vi "Read Output Till Keyword.vi"(7 "timeout [ms]":u32, 8 "error in":errorcluster, 10 "keywords":string[](array[string])=["error", "USERkeyword"], 11 "GOLPI ref. in":T1={"pipe handle"={"lv_proc.dll file path"=path "", "process instance handle"=[]}, "fast read timeout [ms]"=500, "fast read settle time [ms]"=10, "fast read to multiple [ms]"=1, "max elements per input line"=100, "slow read timeout [ms]"=500}) -> (0 "error out":errorcluster, 2 "read buffer":string, 3 "GOLPI ref. out":T1={"pipe handle"={"lv_proc.dll file path"=path "", "process instance handle"=[]}, "fast read timeout [ms]"=500, "fast read settle time [ms]"=10, "fast read to multiple [ms]"=1, "max elements per input line"=100, "slow read timeout [ms]"=500}, 5 "bytes remaining":i32)   [LabVIEW 2013, in "GOLPI library.lvlib"]
doc: "Continually reads output of GNU Octave. If one of strings specified in keywords terminal is found in output, reading stops.\nIf timeout is exceeded, returns only part of buffer and returns number of bytes remaining in the stdout (if any).\nOne of keywords should be 'error' in the case error occurs, otherwise the vi will wait till timeout."
uses:
  GOLPI library.lvlib
  Private/Type Definitions/GOLPI reference Type Def.ctl
  LV Process.lvlibp/Pipe Handle.ctl
  Private/Type Definitions/Custom Error Codes Enum Type Def.vi
  LV Process.lvlibp
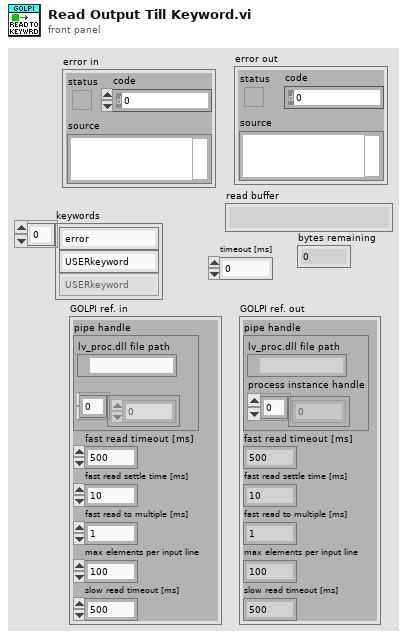
[diagram p1: front panel]
types:
  T1 = typedef "GOLPI library.lvlib/GOLPI reference Type Def.ctl" = cluster{"pipe handle":T2, "fast read timeout [ms]":u32, "fast read settle time [ms]":u32, "fast read to multiple [ms]":u32, "max elements per input line":u32, "slow read timeout [ms]":u32}
  T2 = typedef "LV Process.lvlibp/Pipe Handle.ctl" = cluster{"lv_proc.dll file path":path, "process instance handle":u32[]}
  T3 = typedef "GOLPI library.lvlib/Custom Error Codes Enum Type Def.vi" = enum16{"no error", "00 working directory PAR1 missing", "01 octave binary PAR1 missing", "02 octave report error PAR1", "03 empty output last cmd PAR1", "04 missing temporary file PAR1", "05 pwd PAR 1 not exist", "10 var PAR1 not string", "11 var PAR1 not num, scal, ~compl", "12 var PAR1 not num, scal, compl", "13 var PAR1 not num, vect, ~compl", "14 var PAR1 not num, vect, compl", "15 var PAR1 not num, mat, ~compl", "16 var PAR1 not num, mat, ~compl", "30 WARNING read timeout", "99 not finished"}
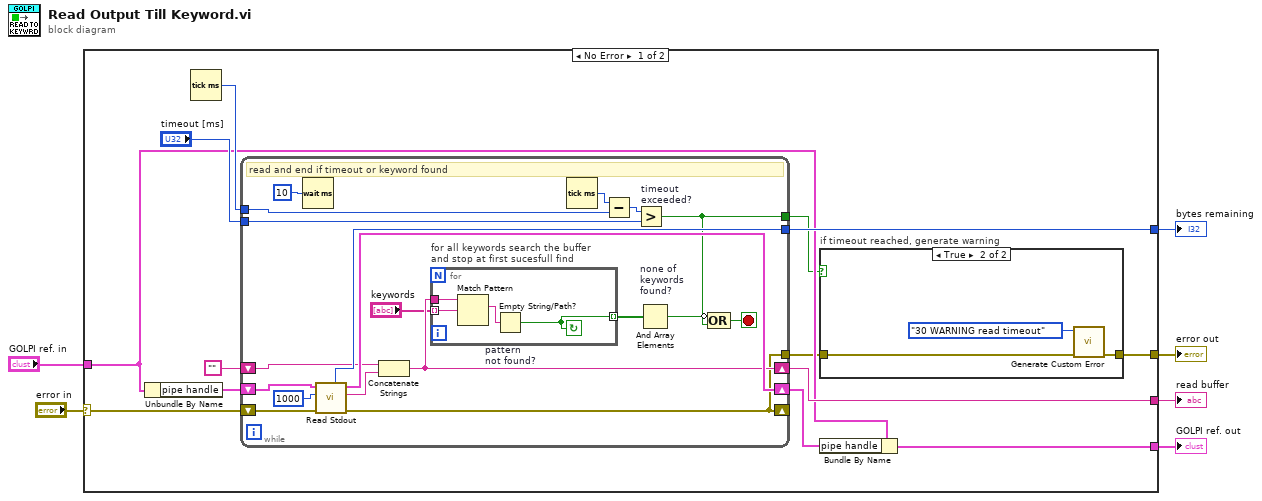
[diagram p0: block diagram]
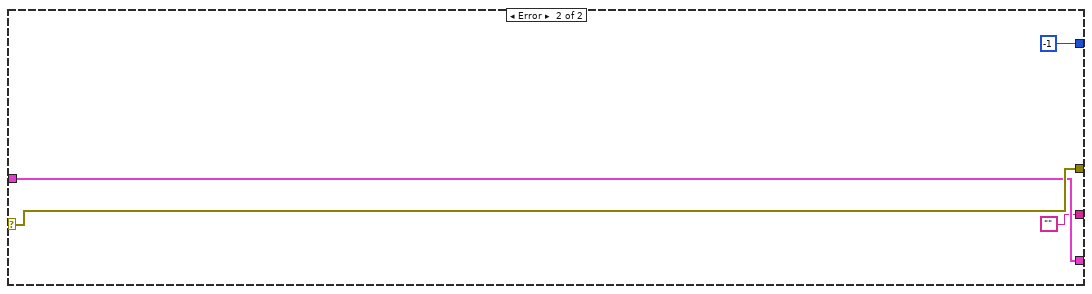
[diagram p3: hidden frame]
diagram:
  n1 = case shown="No Error" "error in" {
    selector: "error in" -> [w7 w50]
    tunnel: [w19 ""] -> w6
    tunnel: [w18 -1 ("bytes remaining")] -> w5
    tunnel: "GOLPI ref. in" -> [w14 w49]
    tunnel: [w13 w49] -> w3
    tunnel: [w9 w50] -> w2
    frame No Error {
      n2 = Unbundle By Name(w14) -> ("pipe handle"=w11:T2)
      n3 = Tick Count (ms)() -> (millisecond timer value=w15:u32)
      n4 = while {
        tunnel: [w36] -> w18
        shift-right: [w41] -> w12
        shift-left: w11 -> [w42]
        shift-right: [w30] -> w19
        shift-left: "" -> [w32]
        tunnel: w15 -> [w39]
        tunnel: "timeout [ms]" -> [w37]
        shift-right: [w25] -> _
        shift-left: w7 -> [w40]
        tunnel: [w25] -> w10
        tunnel: [w24] -> w8
        stop <- w35 stop-if-true
        # "read and end if timeout or keyword found"
        n5 = Wait (ms)(milliseconds to wait=u32 10) -> ()  [unwired: 1 out]
        n6 = call "Read Stdout.vi"("error in"=w40, "byte count"=1000, "pipe in"=w42) -> ("error out"=w25:errorcluster, "read buffer"=w26:string, "pipe out"=w41:T2, "bytes remaining"=w36:i32)  [unwired: 3 in, 2 out]
        n7 = Concatenate Strings(w32, w26) -> (w30:string)
        n8 = for "for all keywords search the buffer\nand stop at first sucesfull find" {
          tunnel: w30 -> [w46]
          tunnel: "keywords" -> [w45] mode=indexing
          tunnel: [w43] -> w28 mode=indexing
          stop <- w43 continue-if-true
          n9 = Match Pattern(string=w46, regular expression=w45) -> (match substring=w44:string)  [unwired: 1 in, 3 out]
          n10 = Empty String/Path? "pattern\nnot found?"(string/path=w44) -> (empty?=w43:bool)
        }
        n11 = Tick Count (ms)() -> (millisecond timer value=w31:u32)
        n12 = Subtract(x=w31, y=w39) -> (x-y=w38:u32)
        n13 = Greater? "timeout\nexceeded?"(x=w38, y=w37) -> (0:w24:bool)
        n14 = And Array Elements "none of\nkeywords\nfound?"(Boolean array=w28) -> (logical AND=w27:bool)
        n15 = Compound Arithmetic op=OR(invert w27, w24) -> (w35:bool)
      }
      n16 = case "if timeout reached, generate warning" shown="True" w8 {
        tunnel: [w20 w21] -> w9
        tunnel: w10 -> [w20 w22]
        frame False {
        }
        frame True {
          n17 = call "Generate Custom Error.vi"("error in"=w22, "GOLPI error"=Custom_Error_Codes_Enum_Type_Def.vi."30 WARNING read timeout") -> ("error out"=w21:errorcluster)  [unwired: 9 in]
        }
      }
      n18 = Bundle By Name(cluster=w14, "pipe handle"=w12) -> (w13:T1)
    }
    frame Error {
    }
  }
  "error out" <- w2
  "read buffer" <- w6
  "bytes remaining" <- w5
  "GOLPI ref. out" <- w3
